vi "Load Sequence.vi"() -> (2 "SEQ out":refnum<class "SEQ.lvclass">)   [LabVIEW 2016, in "Controller.lvlib" / "gController.lvclass"]
uses:
  gController.lvclass
  <vilib>/MSR Consulting, LLC/General Reuse/Sequence/SEQ/SEQ.lvclass
  <vilib>/MSR Consulting, LLC/General Reuse/Sequence/STEPS/STEP.lvclass
  Sequence/O3 Valve Step/O3 Valve Step.lvclass
  C:/Program Files (x86)/National Instruments/LabVIEW 2016/vi.lib/MSR Consulting, LLC/General Reuse/Sequence/STEPS/STEP.lvclass
  Sequence/O2 Valve Step/O2 Valve Step.lvclass
  Sequence/Filter Step/Filter Step.lvclass
  Sequence/UV Power Step/UV Power Step.lvclass
  Sequence/Wait Step/Wait Step.lvclass
  Sequence/Speaker Step/Speaker Step.lvclass
  Sequence/O3 Flow Rate Step/O3 Flow Rate Step.lvclass
  <vilib>/regexp/Match Regular Expression.xnode
panel:
  out "Array":refnum<class "STEP.lvclass">[](array[class])
  in  "seq_path":path=path "c:/cfg/sequence.xml"
  in  "error in":errorcluster
  out "Vals":string[](array[string])
  out "tags":string[](array[string])
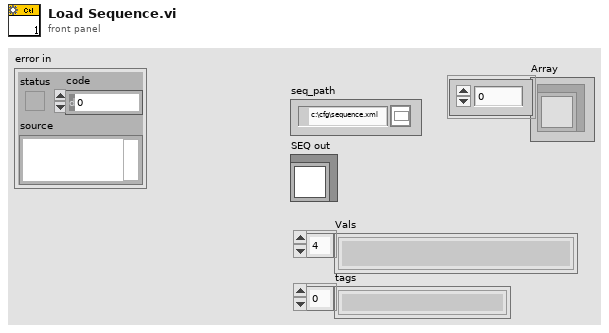
[diagram p1: front panel]
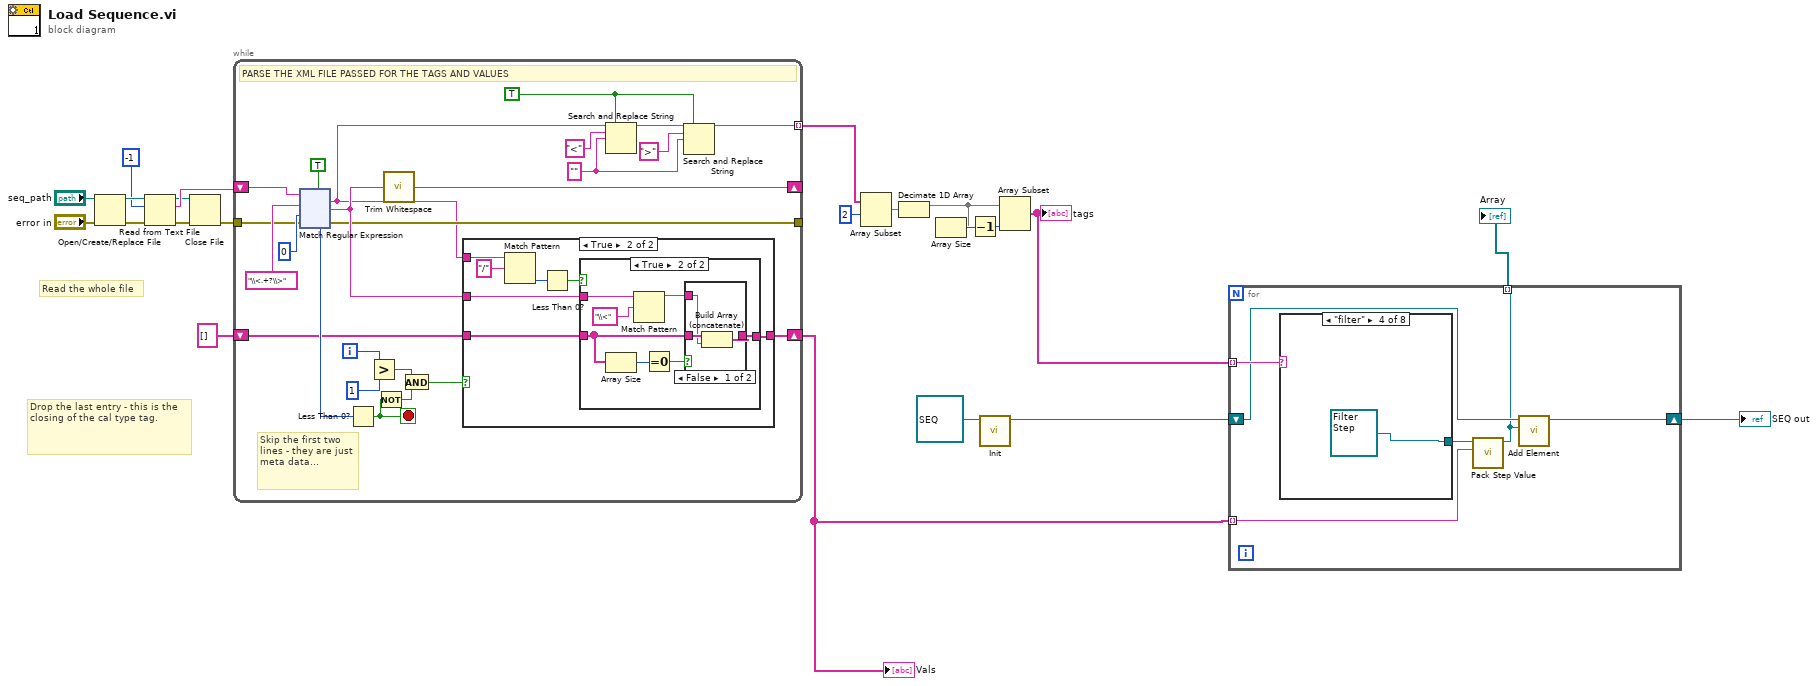
[diagram p0: block diagram]
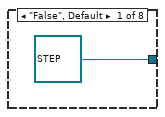
[diagram p2: hidden frame]
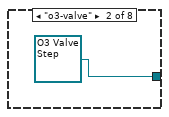
[diagram p3: hidden frame]
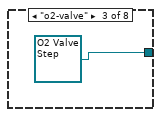
[diagram p4: hidden frame]
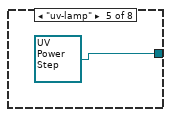
[diagram p5: hidden frame]
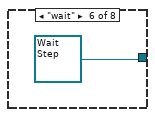
[diagram p6: hidden frame]
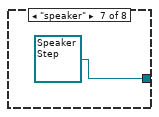
[diagram p7: hidden frame]
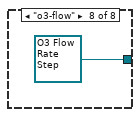
[diagram p8: hidden frame]
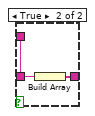
[diagram p11: hidden frame]
diagram:
  # "Read the whole file"
  # "Drop the last entry - this is the closing of the cal type tag."
  n1 = Open/Create/Replace File(file path (use dialog)="seq_path", error in="error in") -> (refnum out=w10:refnum<file>, error out=w11:errorcluster)  [unwired: 4 in, 1 out]
  n2 = Read from Text File(file (use dialog)=w10, count=-1, error in=w11) -> (refnum out=w12:refnum<file>, text=w13:string, error out=w20:errorcluster)  [unwired: 1 in, 1 out]
  n3 = Close File(refnum=w12, error in=w20) -> (error out=w21:errorcluster)  [unwired: 1 out]
  n4 = while {
    shift-right: [w45] -> _
    shift-left: w13 -> [w44]
    shift-right: [w34] -> w3
    shift-left: string[] [] -> [w35]
    tunnel: w21 -> [w31]
    tunnel: [w30] -> _
    tunnel: [w26] -> w22 mode=indexing
    i -> [w39]
    stop <- w32 stop-if-true
    w23 = "" ("replace string (\"\")")
    w25 = TRUE ("ignore case? (F)")
    # "Skip the first two lines - they are just meta data..."
    # "PARSE THE XML FILE PASSED FOR THE TAGS AND VALUES"
    n5 = xnode "Match Regular Expression"("input string"=w44, "regular expression"="\\<.+?\\>", "offset (0)"=0, "error in"=w31, "multiline? (F)"=TRUE) -> ("whole match"=w29:string, "after match"=w41:string, "offset past match"=w42:i32, "error out"=w30:errorcluster)  [unwired: 1 in, 1 out]
    n6 = Less Than 0?(x=w42) -> (x < 0?=w32:bool)
    n7 = Greater?(x=w39, y=1) -> (0:w37:bool)
    n8 = Not(x=w32) -> (.not. x?=w33:bool)
    n9 = call <vilib>:"Trim Whitespace.vi"("string"=w41) -> ("trimmed string"=w45:string)  [unwired: 1 in]
    n10 = And(x=w37, y=w33) -> (x .and. y?=w36:bool)
    n11 = case shown="True" w36 {
      tunnel: w29 -> [_ w54]
      tunnel: w41 -> [_ w50]
      tunnel: w35 -> [w47 w49]
      tunnel: [w47 w48] -> w34
      frame False {
      }
      frame True {
        n12 = Match Pattern(string=w54, regular expression="/") -> (offset past match=w52:i32)  [unwired: 1 in, 3 out]
        n13 = Less Than 0?(x=w52) -> (x < 0?=w51:bool)
        n14 = case shown="True" w51 {
          tunnel: w50 -> [_ w62]
          tunnel: w49 -> [w55 w57]
          tunnel: [w55 w58] -> w48
          frame False {
          }
          frame True {
            n15 = Array Size(array=w57) -> (size(s)=w59:i32)
            n16 = Match Pattern(string=w62, regular expression="\\<") -> (before substring=w56:string)  [unwired: 1 in, 3 out]
            n17 = Equal To 0?(x=w59) -> (x = 0?=w60:bool)
            n18 = case shown="False" w60 {
              tunnel: w56 -> [w63 w67]
              tunnel: [w64 w66] -> w58
              tunnel: w57 -> [w65 _]
              frame False {
                n19 = Build Array (concatenate)(w65, w63) -> (w64:string[])
              }
              frame True {
                n20 = Build Array(w67) -> (w66:string[])
              }
            }
          }
        }
      }
    }
    n21 = Search and Replace String(replace all?=w25, input string=w29, search string="<", replace string=w23) -> (result string=w27:string)  [unwired: 4 in, 3 out]
    n22 = Search and Replace String(replace all?=w25, input string=w27, search string=">", replace string=w23) -> (result string=w26:string)  [unwired: 4 in, 3 out]
  }
  "Vals" <- w3
  n23 = Array Subset(array=w22, index=2) -> (w16:string[])  [unwired: 1 in]
  n24 = Decimate 1D Array(w16) -> (w17:string[])  [unwired: 1 out]
  n25 = Array Size(array=w17) -> (size(s)=w18:i32)
  n26 = Decrement(x=w18) -> (x-1=w19:i32)
  n27 = call-dynamic "Init.vi"("SEQ in"=refnum<class "SEQ.lvclass"> refnum ("Sequence Composition:SEQ")) -> ("SEQ out"=w4:refnum<class "SEQ.lvclass">)  [unwired: 9 in, 1 out]
  n28 = Array Subset(array=w17, length=w19) -> (w5:string[])  [unwired: 1 in]
  "tags" <- w5
  n29 = for {
    tunnel: w5 -> [w187] mode=indexing
    shift-right: [w184] -> w2
    shift-left: w4 -> [w183]
    tunnel: w3 -> [w185] mode=indexing
    tunnel: [w182] -> w1 mode=indexing
    n30 = case shown="\"filter\"" w187 {
      tunnel: [refnum<class "STEP.lvclass"> refnum ("Sequence Composition:STEP.lvclass") refnum<class "O3 Valve Step.lvclass"> refnum ("Controller.lvlib:O3 Valve Step") refnum<class "O2 Valve Step.lvclass"> refnum ("Controller.lvlib:O3 Valve Step") refnum<class "Filter Step.lvclass"> refnum ("Controller.lvlib:Filter Step") refnum<class "UV Power Step.lvclass"> refnum ("Controller.lvlib:O2 Valve Step") refnum<class "Wait Step.lvclass"> refnum ("Controller.lvlib:Wait Step") refnum<class "Speaker Step.lvclass"> refnum ("Controller.lvlib:UV Power Step") refnum<class "O3 Flow Rate Step.lvclass"> refnum ("Controller.lvlib:O3 Flow Rate Step.lvclass")] -> w186
      frame "False", Default {
      }
      frame "o3-valve" {
      }
      frame "o2-valve" {
      }
      frame "filter" {
      }
      frame "uv-lamp" {
      }
      frame "wait" {
      }
      frame "speaker" {
      }
      frame "o3-flow" {
      }
    }
    n31 = call-dynamic "Pack Step Value.vi"("Value"=w185, "STEP in"=w186) -> ("STEP out"=w182:refnum<class "STEP.lvclass">)  [unwired: 8 in, 1 out]
    n32 = call <vilib>:"Add Element.vi"("STEP"=w182, "SEQ in"=w183) -> ("SEQ out"=w184:refnum<class "SEQ.lvclass">)  [unwired: 8 in, 1 out]
  }
  "SEQ out" <- w2
  "Array" <- w1
